vi "AutoLin Anpassung FT-IR.vi"(0 "Eingabetabelle":T3, 5 "Aktiv":T1, 7 "Lin-Polynom":T4 {"zusätzliche Zeitdauer Erster Punkt" format="%#_5g"; "Lin Modus" items=["Cal Gas to PNS", "Cal Gas to Samplepoint", "Measure"]; "Gas Ablaufdatum" format="%<%d.%m.%Y>T"; "HovaCAL Flow AutoLin"."HovaCAL Flow Input Cluster" format="%.2f"; "Gasflasche" items=["----"=10000, "IAG MG"=0, "IAG NH3 3000"=1, "IAG NH3 2000"=2, "IAG NH3 200"=3]; "Conditions:" items=["field", "laboratory"]; "Kalibrierauswahl" items=["Inaktiv", "Aktiv"]; "Anzahl Stufen" format="%#_5g"; "Zeitdauer Stufe" format="%#_5g"; "Verdünnungsgas" items=["N2", "O2"]; "Komponentenauswahl"."Konzentration" format="%#.6f"; "Gasnummer:" min=1 max=5; "Prüfgas Konzentration" format="%#.6f"; "Polynomkoeff." format="%#_18f"}, 9 "Polynom-Ordnung":i32, 11 "error in (no error)":errorcluster caption="Fehler (Eingang, kein Fehler)", 12 "Index (Seite)":i32, 13 "Sprachliste":string[][](array[string])) -> (2 "Ergebnis Lin":string[][](array[string]), 4 "Tabelle":T3, 10 "Lin-Polynom":T4 {"zusätzliche Zeitdauer Erster Punkt" format="%#_5g"; "Lin Modus" items=["Cal Gas to PNS", "Cal Gas to Samplepoint", "Measure"]; "Gas Ablaufdatum" format="%<%d.%m.%Y>T"; "HovaCAL Flow AutoLin"."HovaCAL Flow Input Cluster" format="%.2f"; "Gasflasche" items=["----"=10000, "IAG MG"=0, "IAG NH3 3000"=1, "IAG NH3 2000"=2, "IAG NH3 200"=3]; "Conditions:" items=["field", "laboratory"]; "Kalibrierauswahl" items=["Inaktiv", "Aktiv"]; "Anzahl Stufen" format="%#_5g"; "Zeitdauer Stufe" format="%#_5g"; "Verdünnungsgas" items=["N2", "O2"]; "Komponentenauswahl"."Konzentration" format="%#.6f"; "Gasnummer:" min=1 max=5; "Prüfgas Konzentration" format="%#.6f"; "Polynomkoeff." format="%#_18f"}, 15 "error out":errorcluster caption="Fehler (Ausgang)")   [LabVIEW 2020, in "Linearisierung v2.lvlib"]
doc: "Berechnet die Polynomkoeffizienten, die zur Linearisierung beliebiger Messdaten (Rohwerte) notwendig sind, aus einem 2D-Array mit N Konzentrationswerten in ppm\n 1. Spalte: Gasteiler (Kalibriervorgabe)\n 2. Spalte: Messgerät\nunter Vorgabe eines maximal erlaubten Fehlers in % vom Endwert (Gasteiler).\n\nWenn die Polynom-Ordnung mit Null (Standardwert) vorgewählt wird, wird die kleinste Ordnung ermittelt, die den erlaubten Fehler unterschreitet und die Polynomanpassung damit durchgeführt.\nWenn eine Polynom-Ordnung von 1 bis 4 gewählt wird, erfolgt die Anpassung mit der gewünschten Ordnung.\n\nAusgabe \"Lin-Polynom\", Cluster aus:\n\"F_max gefordert (%)\":\ngeforderte Genauigkeit der Polynomanpassung, bezogen auf Endwert (Gasteiler)\n\n\"F_max in %\":\ngrößte Abweichung der linearisierten Messdaten von den Sollwerten in % bezogen auf den Endwert (Gasteiler)\n\n\"F_max in ppm\":\ngrößte Abweichung der linearisierten Messdaten von den Sollwerten in ppm\n\n\"Vorschlag Ordnung\":\ngewählte Polynomordnung bei automatischer Verarbeitung, 0 bei manueller Wahl der Ordnung\n\n\"Polynom OK\"\nTRUE wenn der vorgegebene maximale Fehler unterschritten wurde\n\n\"Polynomkoeff.\":\ndirekt verwendbar zur Polynom-Entwicklung mit dem polymorphen VI \"polynomial evaluation\" (skalare, 1D oder 2D-Daten)."
uses:
  Linearisierung v2.lvlib
  Eingabetabelle.ctl
  Lin-Polynom Daten.ctl
  KomponentenArray.ctl
  Visualisierungs Elemente/Auswahlfeld.ctl
  Visualisierungs Elemente/Zahlen-Eingabefeld.ctl
  EPA Optionsfeld.ctl
  Gasteiler/HovaCal/AutoLin Hovacal.ctl
  Kalibrieroption.ctl
  EPA1065-307/Condition.ctl
  Seiten/System Einstellungen V2/Konfig Gasflasche.ctl
  Seiten/System Einstellungen V2/Gasflasche Auswahl.ctl
  Gasteiler/HovaCAL_Interface/Controls/Flow Einstellung.ctl
  Gasteiler/HovaCAL_Interface/Controls/Pump state.ctl
  Seiten/CalGas Aufschaltung/Lin Modus.ctl
  AktivArray.ctl
  AktivButton.ctl
  <vilib>/Analysis/6fits.llb/Curve Fitting Criteria.ctl
  Aktionen Polynom Daten speichern.ctl
  <vilib>/Analysis/NI_AALPro.lvlib
  AutoLin Protokoll/AutoLin Protokoll.lvlib
  Gasteiler/Gasteiler.lvlib
  Gasteiler/HovaCal/HovaCal.lvlib
  EPA1065-307/Linearity verification 1065-307.lvlib
  Seiten/System Einstellungen V2/System Einstellungen V2.lvlib
  Gasteiler/HovaCAL_Interface/Controls/Controls.lvlib
  Seiten/CalGas Aufschaltung/CalGas Aufschaltung.lvlib
panel:
  out "XY-Graph (roh/lin)":cluster{"eine Kurve":sgl[], dbl[]}[](array[cluster])
  # "Messgerät (ppm)"
  # "Gasteiler (ppm)"
  # "Tabelle:\n0.....Sollwert\n1.....Istwert\n2.....Rohwert\n3.....linearisiert\n4.....abs.Fehler ppm\n5.....Fehler in %\n6.....Deviation\n7.....Temp.Messzelle\n8.....Druck Messzelle\n9.....abs.Fehler ppm linearisiert\n10....Fehler in % linearisiert\n11....abs.Fehler ppm EPA\n12....Fehler in % EPA\n13....abs.Fehler ppm Rohwert\n14....Fehler in % Rohwert"
  # "%"
  # "%"
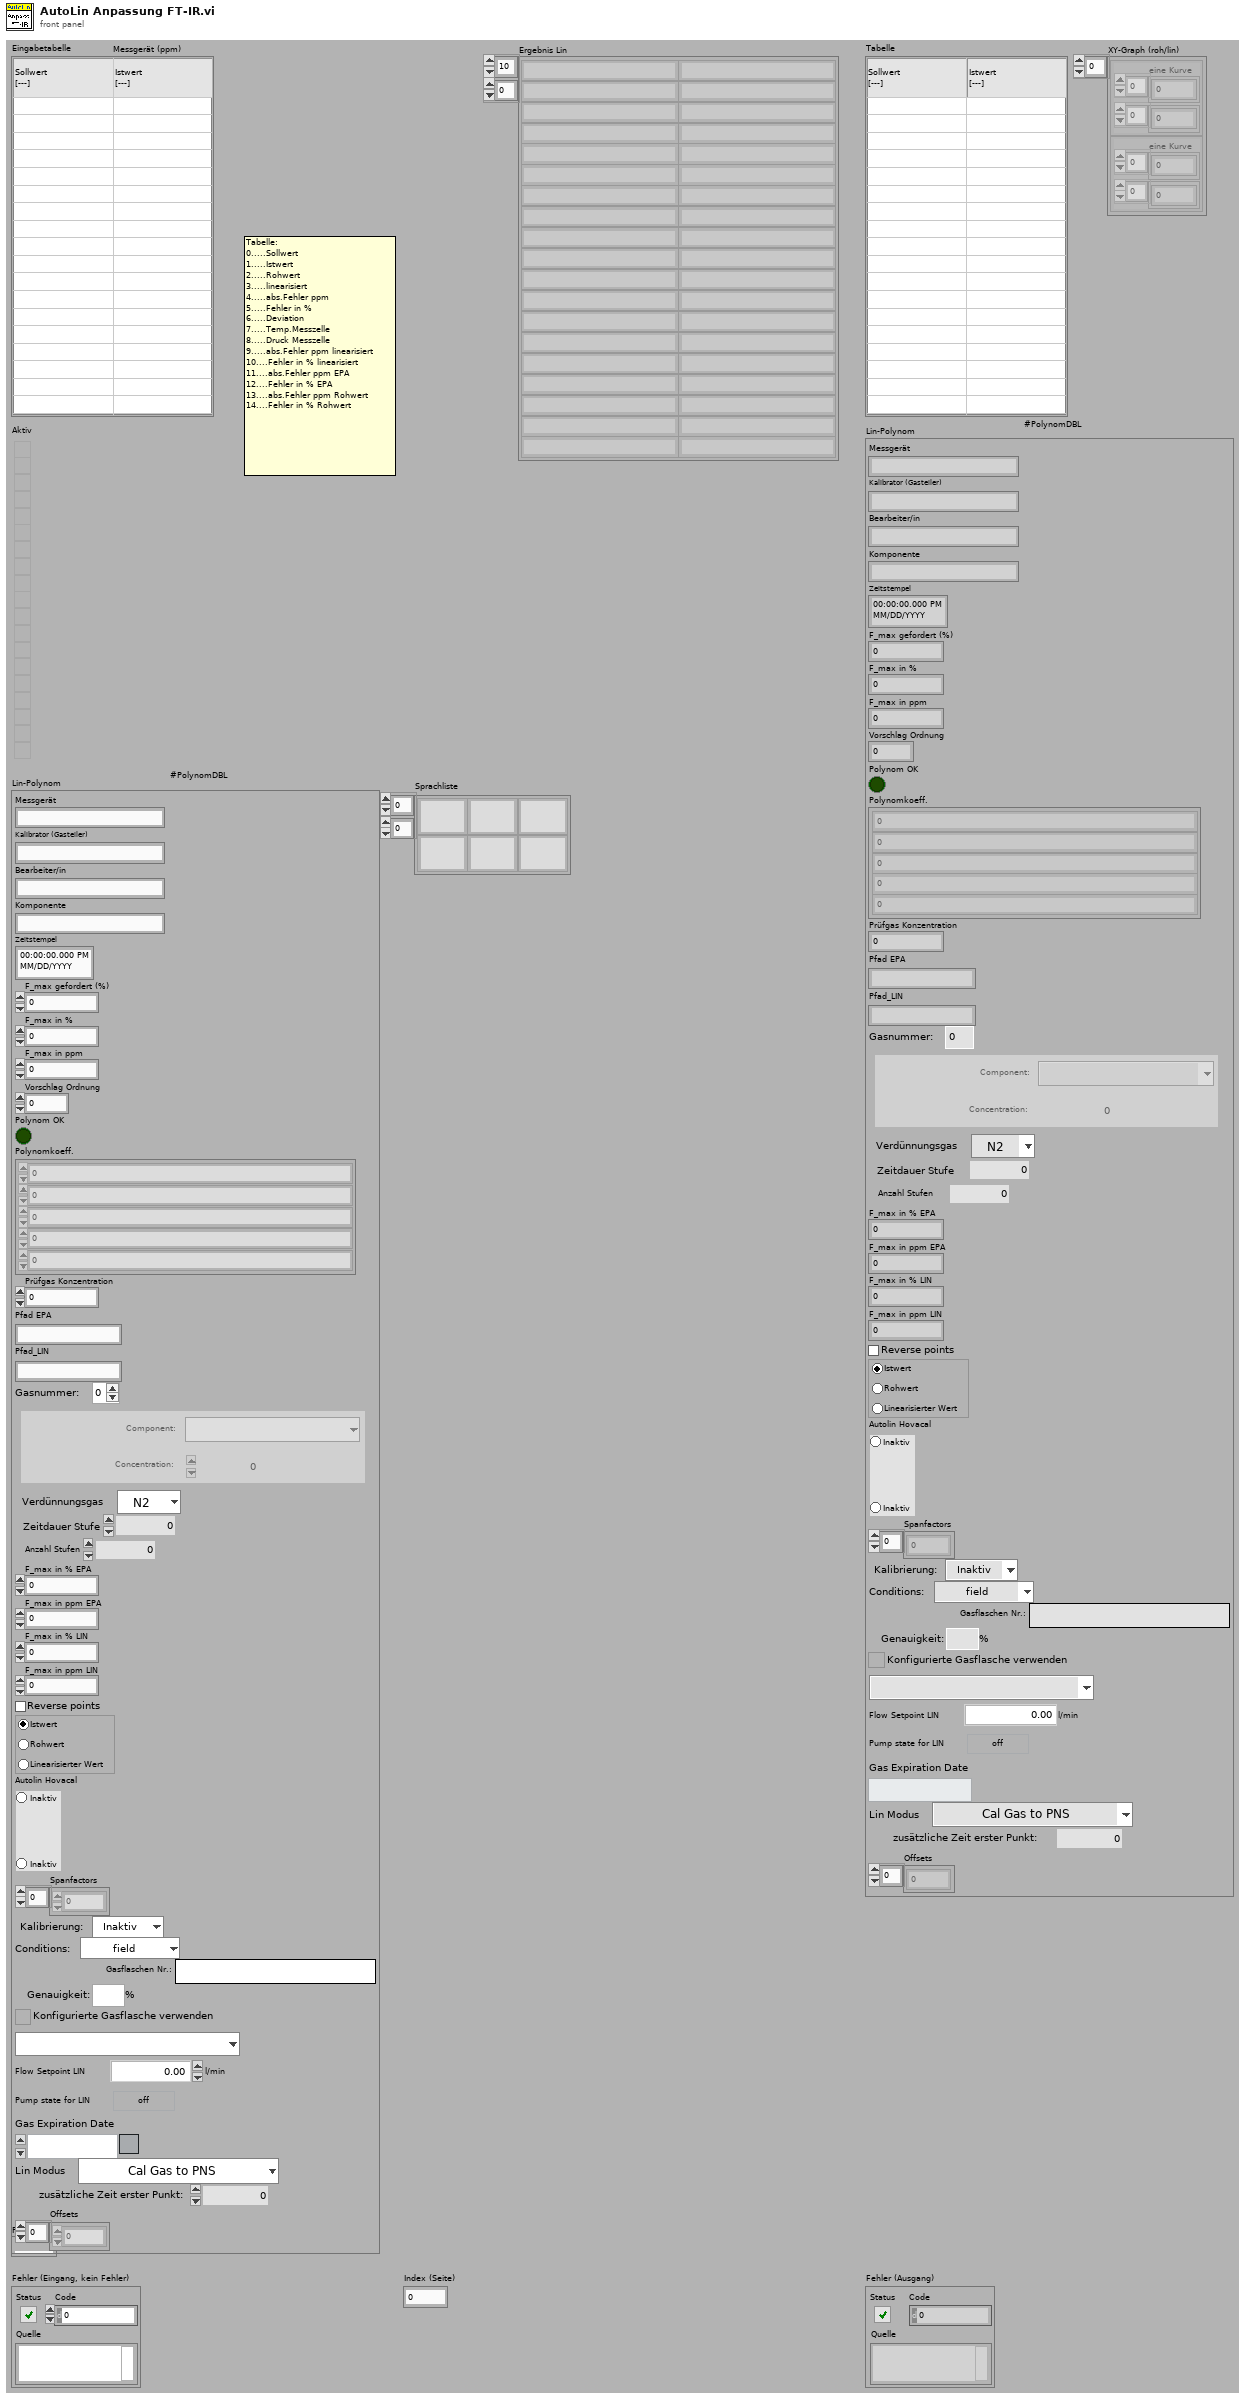
[diagram p1: front panel]
types:
  T1 = typedef "Linearisierung v2.lvlib/AktivArray.ctl" = T2[]
  T2 = typedef "Linearisierung v2.lvlib/AktivButton.ctl" = bool
  T3 = typedef "Linearisierung v2.lvlib/Eingabetabelle.ctl" = string[][]
  T4 = typedef "Linearisierung v2.lvlib/Lin-Polynom Daten.ctl" = cluster{"Messgerät":string, "Kalibrator (Gasteiler)":string, "Bearbeiter/in":string, "Komponente":string, "Zeitstempel":timestamp, "F_max gefordert (%)":sgl, "F_max in %":sgl, "F_max in ppm":sgl, "Vorschlag Ordnung":i32, "Polynom OK":bool, "Polynomkoeff.":dbl[], "Prüfgas Konzentration":dbl, "Pfad EPA":string, "Pfad_LIN":string, "Gasnummer:":u8, "Komponentenauswahl":T5, "Verdünnungsgas":T7, "Zeitdauer Stufe":T8, "Anzahl Stufen":T8, "F_max in % EPA":sgl, "F_max in ppm EPA":sgl, "F_max in % LIN":sgl, "F_max in ppm LIN":sgl, "Punkte umkehren":bool, "EPA Optionsfeld":T9, "Autolin Hovacal":T10, "Spanfactors":sgl[], "Kalibrierauswahl":T11, "Conditions:":T12, "Gasflaschen Nr.:":string, "Bottle Accuracy":dbl, "Konfig Gasflasche":T13, "Gasflasche":T14, "HovaCAL Flow AutoLin":T15, "MFC Output":T16, "Gas Ablaufdatum":timestamp, "Lin Modus":T17, "zusätzliche Zeitdauer Erster Punkt":sgl, "Offsets":sgl[]}
  T5 = typedef "Linearisierung v2.lvlib/KomponentenArray.ctl" = cluster{"Komponente:":T6, "Konzentration":dbl}[]
  T6 = typedef "Auswahlfeld.ctl" = u16
  T7 = typedef "Linearisierung v2.lvlib/Gasteiler.lvlib/Prüfgas in.ctl" = u16
  T8 = typedef "Zahlen-Eingabefeld.ctl" = sgl
  T9 = typedef "Linearisierung v2.lvlib/EPA Optionsfeld.ctl" = enum32{"Istwert", "Rohwert", "Linearisierter Wert"}
  T10 = typedef "Linearisierung v2.lvlib/Gasteiler.lvlib/HovaCal.lvlib/AutoLin Hovacal.ctl" = enum32{"Keine Auswahl", "Optionsauswahl 1", "Optionsauswahl 2"}
  T11 = typedef "Linearisierung v2.lvlib/Kalibrieroption.ctl" = u16
  T12 = typedef "Linearisierung v2.lvlib/Linearity verification 1065-307.lvlib/Condition.ctl" = u16
  T13 = typedef "System Einstellungen V2.lvlib/Konfig Gasflasche.ctl" = bool
  T14 = typedef "System Einstellungen V2.lvlib/Gasflasche Auswahl.ctl" = u16
  T15 = typedef "Linearisierung v2.lvlib/Gasteiler.lvlib/HovaCAL_Interface.lvlib/Controls.lvlib/Flow Einstellung.ctl" = cluster{"HovaCAL Flow Input Cluster":dbl}
  T16 = typedef "Linearisierung v2.lvlib/Gasteiler.lvlib/HovaCAL_Interface.lvlib/Controls.lvlib/Pump state.ctl" = cluster{"Run":bool}
  T17 = typedef "CalGas Aufschaltung.lvlib/Lin Modus.ctl" = u16
  T18 = typedef "Linearisierung v2.lvlib/Aktionen Polynom Daten speichern.ctl" = enum16{"lesen", "laden", "speichern", "schreiben", "schreiben alle", "Liste erstellen", "aktivieren", "deaktivieren", "aktiv abfragen"}
  T19 = typedef "NI_AALPro.lvlib/Curve Fitting Criteria.ctl" = u16
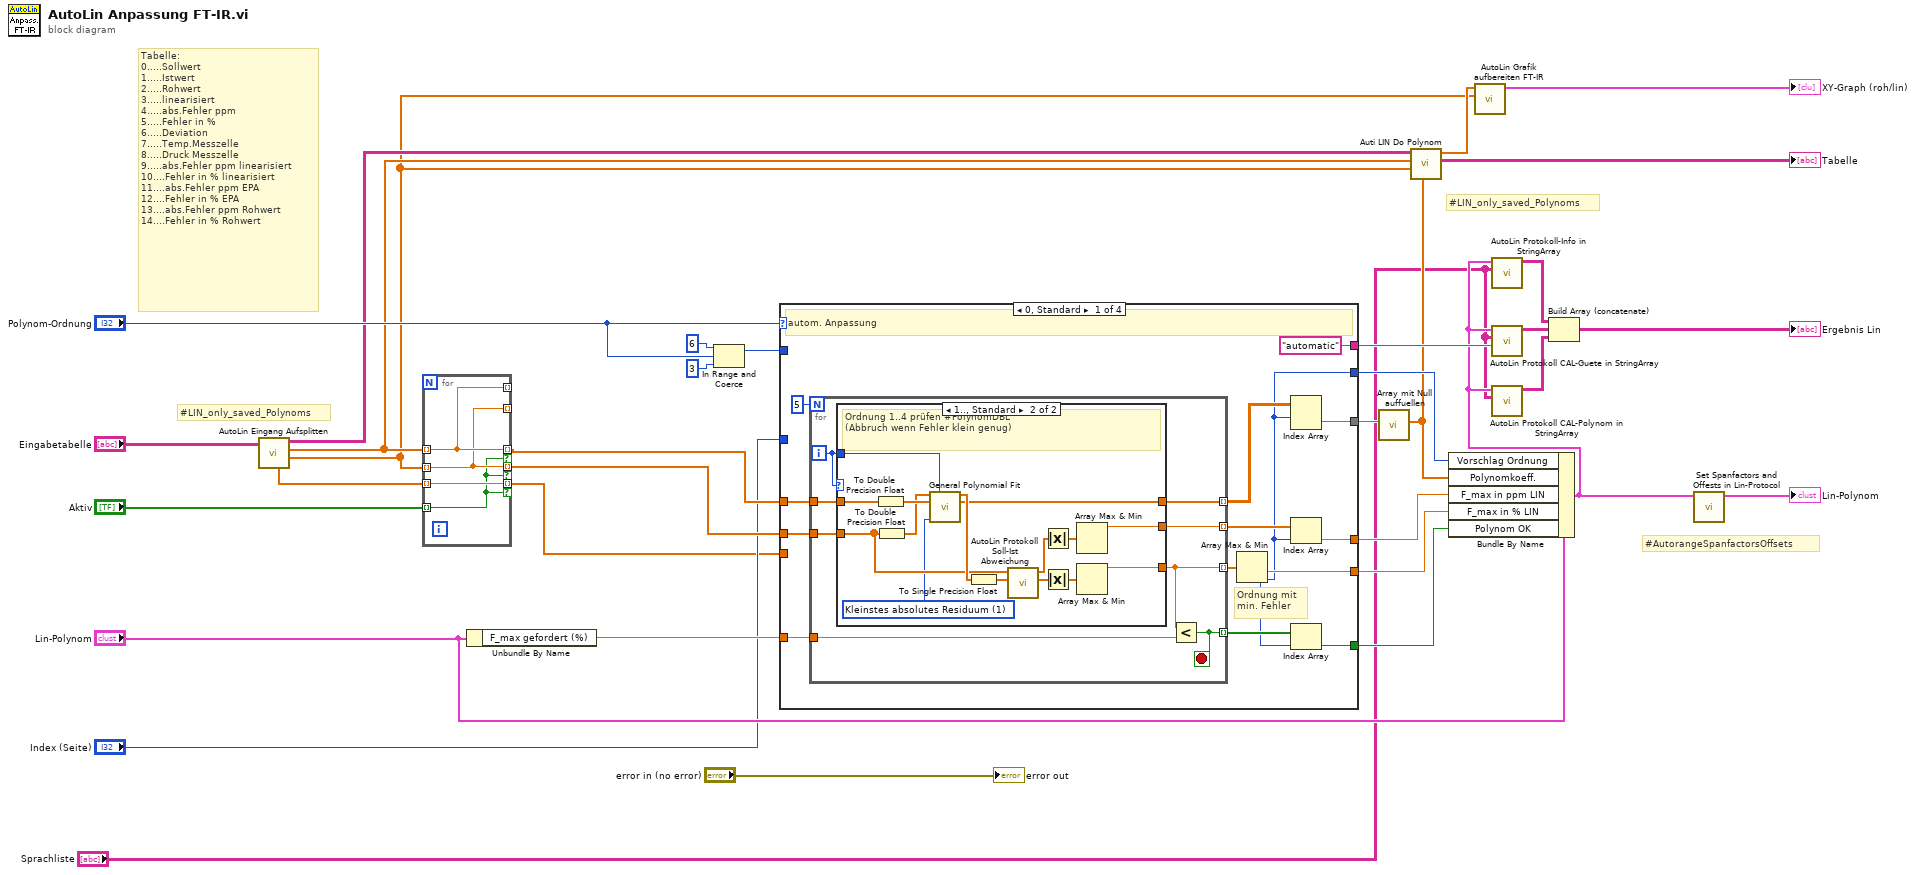
[diagram p0: block diagram]
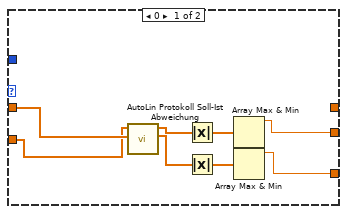
[diagram p2: hidden frame]
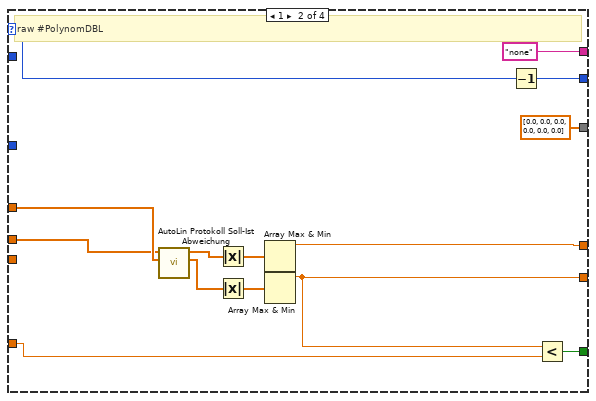
[diagram p3: hidden frame]
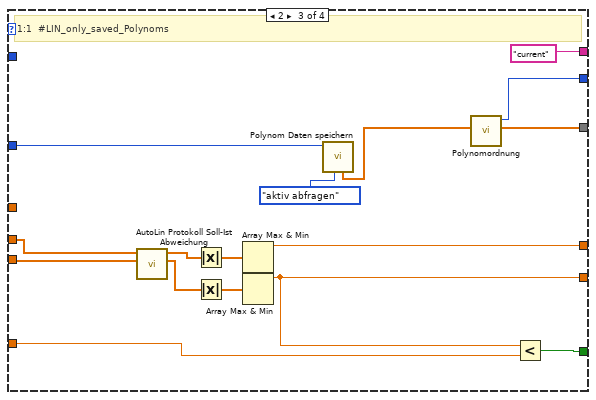
[diagram p4: hidden frame]
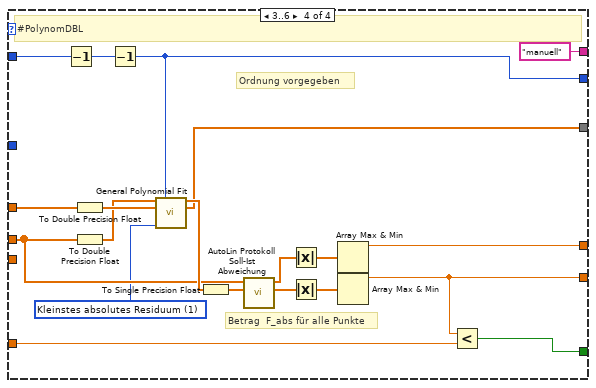
[diagram p5: hidden frame]
diagram:
  # "#LIN_only_saved_Polynoms"
  # "#LIN_only_saved_Polynoms"
  # "#AutorangeSpanfactorsOffsets"
  # "Tabelle:\n0.....Sollwert\n1.....Istwert\n2.....Rohwert\n3.....linearisiert\n4.....abs.Fehler ppm\n5.....Fehler in %\n6.....Deviation\n7.....Temp.Messzelle\n8.....Druck Messzelle\n9.....abs.Fehler ppm linearisiert\n10....Fehler in % linearisiert\n11....abs.Fehler ppm EPA\n12....Fehler in % EPA\n13....abs.Fehler ppm Rohwert\n14....Fehler in % Rohwert"
  n1 = call "AutoLin Eingang Aufsplitten.vi"("Eingabetabelle"="Eingabetabelle") -> ("Sollwerte"=w3:dbl[], "Rohwerte"=w4:dbl[], "Eingabetabelle out"=w5:T3, "Linearisiert"=w2:dbl[])  [unwired: 6 in, 1 out]
  n2 = for {
    tunnel: w4 -> [w38] mode=indexing
    tunnel: w3 -> [w37] mode=indexing
    tunnel: [w38] -> w15 mode=indexing if=w35
    tunnel: [w37] -> w14 mode=indexing if=w35
    tunnel: "Aktiv" -> [w35] mode=indexing
    tunnel: [w38] -> _ mode=indexing
    tunnel: [w37] -> _ mode=indexing
    tunnel: [w36] -> w9 mode=indexing if=w35
    tunnel: w2 -> [w36] mode=indexing
  }
  n3 = Unbundle By Name("Lin-Polynom") -> ("F_max gefordert (%)"=w25:sgl)
  n4 = In Range and Coerce(upper limit=6 ("Obergrenze"), x="Polynom-Ordnung", lower limit=3 ("Untergrenze")) -> (coerced(x)=w30:i32)  [unwired: 1 out]
  n5 = case shown="0, Standard" "Polynom-Ordnung" {
    selector: "Polynom-Ordnung" -> [_ w91 _ _]
    tunnel: w15 -> [w52 w97 _ w129]
    tunnel: w14 -> [w51 w96 w103 w124]
    tunnel: w30 -> [_ _ _ w117]
    tunnel: w25 -> [w49 w87 w106 w133]
    tunnel: [w46 dbl[] [0.0, 0.0, 0.0, 0.0, 0.0, 0.0] w101 w125] -> w26
    tunnel: [w48 w86 w104 w131] -> w27
    tunnel: [w44 w88 w107 w130] -> w33
    tunnel: [w41 w90 w100 w116] -> w28
    tunnel: [w40 w89 w105 w120] -> w29
    tunnel: ["automatic" "none" "current" "manuell"] -> w12
    tunnel: "Index (Seite)" -> [_ _ w99 _]
    tunnel: w9 -> [_ _ w102 _]
    frame 0, Default {
      # "Ordnung mit\nmin. Fehler"
      # "autom. Anpassung"
      n6 = for {
        N: 5 -> [_]
        tunnel: w52 -> [w57]
        tunnel: w51 -> [w55]
        tunnel: [w56] -> w47 mode=indexing
        tunnel: w49 -> [w60]
        tunnel: [w58] -> w43 mode=indexing
        tunnel: [w59] -> w45 mode=indexing
        tunnel: [w54] -> w42 mode=indexing
        i -> [w53]
        stop <- w59 stop-if-true
        n7 = case shown="1.., Standard" w53 {
          tunnel: [w63 w82] -> w58
          tunnel: w57 -> [w62 w81]
          tunnel: [_ w77] -> w56
          tunnel: w55 -> [w61 w75]
          tunnel: [w64 w71] -> w54
          tunnel: w53 -> [_ w69]
          frame 0 {
            n8 = call "AutoLin Protokoll Soll-Ist Abweichung.vi"("Istwerte (ppm)"=w62, "Sollwerte (ppm)"=w61) -> ("% vom Sollwert"=w65:sgl[], "abs. Fehler (ppm)"=w66:sgl[])  [unwired: 7 in, 1 out]
            n9 = Absolute Value(x=w66) -> (abs(x)=w68:sgl[])
            n10 = Absolute Value(x=w65) -> (abs(x)=w67:sgl[])
            n11 = Array Max & Min(array=w68) -> (max value=w64:sgl)  [unwired: 3 out]
            n12 = Array Max & Min(array=w67) -> (max value=w63:sgl)  [unwired: 3 out]
          }
          frame 1.., Default {
            w70 = T19 1 items=["Kleinstes Quadrat", "Kleinstes absolutes Residuum", "Biquadrat"] ("method")
            # "Ordnung 1..4 prüfen #PolynomDBL\n(Abbruch wenn Fehler klein genug)"
            n13 = To Double Precision Float(number=w81) -> (double precision float=w80:dbl[])
            n14 = To Double Precision Float(number=w75) -> (double precision float=w79:dbl[])
            n15 = call <vilib>:"General Polynomial Fit.vi"("Y"=w79, "polynomial order"=w69, "X"=w80, "method"=w70) -> ("Best Polynomial Fit"=w78:dbl[], "Polynomial Coefficients"=w77:dbl[])  [unwired: 8 in, 2 out]
            n16 = To Single Precision Float(number=w78) -> (single precision float=w76:sgl[])
            n17 = call "AutoLin Protokoll Soll-Ist Abweichung.vi"("Istwerte (ppm)"=w76, "Sollwerte (ppm)"=w75) -> ("% vom Sollwert"=w74:sgl[], "abs. Fehler (ppm)"=w73:sgl[])  [unwired: 7 in, 1 out]
            n18 = Absolute Value(x=w73) -> (abs(x)=w72:sgl[])
            n19 = Absolute Value(x=w74) -> (abs(x)=w83:sgl[])
            n20 = Array Max & Min(array=w72) -> (max value=w71:sgl)  [unwired: 3 out]
            n21 = Array Max & Min(array=w83) -> (max value=w82:sgl)  [unwired: 3 out]
          }
        }
        n22 = Less?(x=w58, y=w60) -> (x < y?=w59:bool)
      }
      n23 = Array Max & Min(array=w43) -> (min value=w48:sgl, min index (indices)=w41:i32)  [unwired: 2 out]
      n24 = Index Array(array=w47, index (row)=w41) -> (element=w46:dbl[])  [unwired: 1 in]
      n25 = Index Array(array=w42, index=w41) -> (element=w40:sgl)
      n26 = Index Array(array=w45, index=w41) -> (element=w44:bool)
    }
    frame 1 {
      # "raw #PolynomDBL"
      n27 = call "AutoLin Protokoll Soll-Ist Abweichung.vi"("Istwerte (ppm)"=w97, "Sollwerte (ppm)"=w96) -> ("% vom Sollwert"=w92:sgl[], "abs. Fehler (ppm)"=w93:sgl[])  [unwired: 7 in, 1 out]
      n28 = Absolute Value(x=w93) -> (abs(x)=w95:sgl[])
      n29 = Absolute Value(x=w92) -> (abs(x)=w94:sgl[])
      n30 = Array Max & Min(array=w95) -> (max value=w89:sgl)  [unwired: 3 out]
      n31 = Array Max & Min(array=w94) -> (max value=w86:sgl)  [unwired: 3 out]
      n32 = Decrement(x=w91) -> (x-1=w90:i32)
      n33 = Less?(x=w86, y=w87) -> (x < y?=w88:bool)
    }
    frame 2 {
      # "1:1  #LIN_only_saved_Polynoms"
      n34 = call "AutoLin Protokoll Soll-Ist Abweichung.vi"("Istwerte (ppm)"=w102, "Sollwerte (ppm)"=w103) -> ("% vom Sollwert"=w108:sgl[], "abs. Fehler (ppm)"=w109:sgl[])  [unwired: 7 in, 1 out]
      n35 = Absolute Value(x=w109) -> (abs(x)=w111:sgl[])
      n36 = Absolute Value(x=w108) -> (abs(x)=w110:sgl[])
      n37 = Array Max & Min(array=w111) -> (max value=w105:sgl)  [unwired: 3 out]
      n38 = Array Max & Min(array=w110) -> (max value=w104:sgl)  [unwired: 3 out]
      n39 = call "Polynom Daten speichern.vi"("Aktionen"=Aktionen_Polynom_Daten_speichern."aktiv abfragen", "Komponente"=w99) -> ("Einzelnes Polynom out"=w98:dbl[])  [unwired: 4 in, 5 out]
      n40 = call "Polynomordnung.vi"("LIN Polynom"=w98) -> ("LIN Polynom out"=w101:dbl[], "Polynomordnung"=w100:i32)  [unwired: 9 in]
      n41 = Less?(x=w104, y=w106) -> (x < y?=w107:bool)
    }
    frame 3..6 {
      w118 = T19 1 items=["Kleinstes Quadrat", "Kleinstes absolutes Residuum", "Biquadrat"] ("method")
      # "Betrag  F_abs für alle Punkte"
      # "Ordnung vorgegeben"
      # "#PolynomDBL"
      n42 = Decrement(x=w117) -> (x-1=w114:i32)
      n43 = To Double Precision Float(number=w129) -> (double precision float=w128:dbl[])
      n44 = To Double Precision Float(number=w124) -> (double precision float=w127:dbl[])
      n45 = Decrement(x=w114) -> (x-1=w116:i32)
      n46 = call <vilib>:"General Polynomial Fit.vi"("Y"=w127, "polynomial order"=w116, "X"=w128, "method"=w118) -> ("Best Polynomial Fit"=w126:dbl[], "Polynomial Coefficients"=w125:dbl[])  [unwired: 8 in, 2 out]
      n47 = To Single Precision Float(number=w126) -> (single precision float=w123:sgl[])
      n48 = call "AutoLin Protokoll Soll-Ist Abweichung.vi"("Istwerte (ppm)"=w123, "Sollwerte (ppm)"=w124) -> ("% vom Sollwert"=w122:sgl[], "abs. Fehler (ppm)"=w119:sgl[])  [unwired: 7 in, 1 out]
      n49 = Absolute Value(x=w119) -> (abs(x)=w121:sgl[])
      n50 = Absolute Value(x=w122) -> (abs(x)=w132:sgl[])
      n51 = Array Max & Min(array=w121) -> (max value=w120:sgl)  [unwired: 3 out]
      n52 = Array Max & Min(array=w132) -> (max value=w131:sgl)  [unwired: 3 out]
      n53 = Less?(x=w131, y=w133) -> (x < y?=w130:bool)
    }
  }
  n54 = call "Array mit Null auffuellen.vi"("Array"=w26) -> ("Array 2"=w6:dbl[])  [unwired: 10 in]
  n55 = call "Auti LIN Do Polynom.vi"("Polynomkoeff."=w6, "Sollwerte"=w3, "Rohwerte"=w4, "Eingabetabelle"=w5) -> ("Tabelle"=→"Tabelle":string[][], "Linearisiert"=w21:dbl[])  [unwired: 5 in, 1 out]
  n56 = Bundle By Name(cluster="Lin-Polynom", "Vorschlag Ordnung"=w28, "Polynomkoeff."=w6, "F_max in ppm LIN"=w29, "F_max in % LIN"=w27, "Polynom OK"=w33) -> (w7:T4)
  n57 = call "AutoLin Grafik aufbereiten FT-IR.vi"("Sollwerte"=w3, "Istwerte"=w21) -> ("XY-Graph (roh/lin)"=→"XY-Graph (roh/lin)":cluster{"eine Kurve":sgl[], dbl[]}[])  [unwired: 9 in]
  n58 = call "AutoLin Protokoll-Info in StringArray.vi"("Sprachliste"="Sprachliste", "Lin-Polynom"=w7) -> ("Protokoll-Info-String"=w20:string[][])  [unwired: 9 in]
  n59 = call "AutoLin Protokoll CAL-Guete in StringArray.vi"("MAN/AUTO"=w12, "Sprachliste"="Sprachliste", "Lin-Polynom"=w7) -> ("Lin-Güte (Protokoll)"=w19:string[][])  [unwired: 8 in]
  n60 = call "AutoLin Protokoll CAL-Polynom in StringArray.vi"("Sprachliste"="Sprachliste", "Lin-Polynom"=w7) -> ("LinPolynom (Protokoll)"=w18:string[][])  [unwired: 9 in]
  n61 = Build Array (concatenate)(w20, w19, w18) -> (→"Ergebnis Lin":string[][])
  n62 = call "Set Spanfactors and Offests in Lin-Protocol.vi"("Lin-Polynom"=w7) -> ("Lin-Polynom out"=→"Lin-Polynom":T4)  [unwired: 7 in, 3 out]
  "error out" <- "error in (no error)"
